vi "Stop Core.vi"(10 "final error code":i32, 11 "PLC Sim Controller Actor in":refnum<class "PLC Sim Controller Actor.lvclass">) -> (3 "PLC Sim Controller Actor out":refnum<class "PLC Sim Controller Actor.lvclass">)   [LabVIEW 2019, in "PLC Sim Controller Actor.lvlib" / "PLC Sim Controller Actor.lvclass"]
doc: "(<B>Filename</B>: Actor Framework.lvlib:Actor.lvclass:Stop Core.vi)\n\nDefines what the actor does before it stops. Use the <B>final error code</B> input to determine whether the actor shut down in response to an error.\n\nBy default, this method passes the Stop message along to all auto-stop nested actors. A descendant class may override this method to define additional behavior, such as shutting down any processes the actor initiated in its override of the Actor Core method."
uses:
  PLC Sim Controller Actor.lvclass
  PLC Sim Controller Actor.lvclass/PLC Sim Controller Actor.ctl
  <vilib>/ActorFramework/Actor/Actor.lvclass
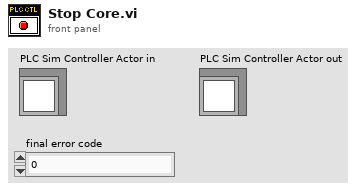
[diagram p1: front panel]
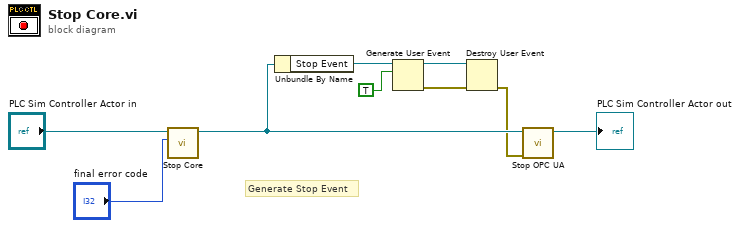
[diagram p0: block diagram]
diagram:
  # "Generate Stop Event"
  n1 = call-parent "Stop Core.vi"("final error code"="final error code", "Actor in"="PLC Sim Controller Actor in") -> ("Actor out"=w3:refnum<class "PLC Sim Controller Actor.lvclass">)  [unwired: 9 in]
  n2 = Unbundle By Name(w3) -> ("Stop Event"=w7:refnum<user-event>)
  n3 = Generate User Event(user event=w7, event data cluster=TRUE ("event data")) -> (user event out=w4:refnum<user-event>, error out=w5:errorcluster)  [unwired: 2 in]
  n4 = Destroy User Event(user event=w4, error in=w5) -> (error out=w1:errorcluster)
  n5 = call "Stop OPC UA.vi"("error in (no error)"=w1, "SM EOL Station Actor in"=w3) -> ("SM EOL Station Actor out"=→"PLC Sim Controller Actor out":refnum<class "PLC Sim Controller Actor.lvclass">)  [unwired: 8 in, 1 out]
